vi "GA_FitnessFunction.vi"(1 "Init? (F)":bool, 2 "ClassifierClass.lvclass":refnum<class "ClassifierClass.lvclass">, 3 "Phenotype":i8[](array[numeric])) -> (0 "Fitness":dbl)   [LabVIEW 2016, in "GA.lvlib"]
uses:
  GA.lvlib
  4. Accuracy Assessment for EEG Classification/_vlib/ClassifierClass.lvclass
  4. Accuracy Assessment for EEG Classification/_vlib/CU_DataTypes.ctl
  4. Accuracy Assessment for EEG Classification/Classifier.lvlib
panel:
  # "This VI is a part of BCI Design library, http://www.ru-bci.org \nCopyright © 2020, Sotnikov Peter, All rights reserved. License: GNU GPLv3"
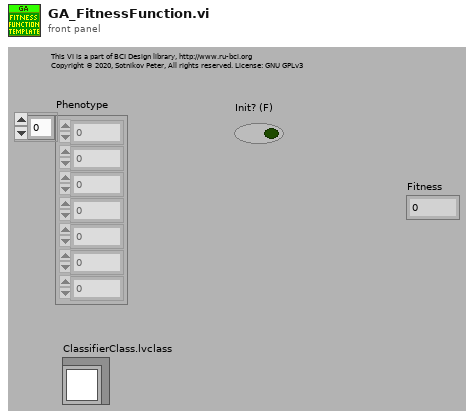
[diagram p1: front panel]
types:
  T1 = typedef "Classifier.lvlib/CU_DataTypes.ctl" = enum16{"Training Data", "Test Data", "Training Data (cross-check)", "Test Data (cross-check)"}
  T2 = typedef "Classifier.lvlib/CU_ClassifierTypes.ctl" = enum16{"Multilayer perceptron", "k NN Classifier", "SVM Committee", "Mahalanobis distance", "SVM Classifier"}
  T3 = typedef "IMAQ Classifier Session.ctl" = refnum<k1>
  T4 = typedef "NILabs_MLT.lvlib/ml_BP_Project.ctl" = cluster{"Training Data":T5, "Normalize Info":T6, "3-layer NN":T7, "Ternimal Condition":T8}
  T5 = typedef "NILabs_MLT.lvlib/ml_BP_Data.ctl" = cluster{"dim in":i32, "dim out":i32, "# samples":i32, "Input":dbl[][], "Output":dbl[][]}
  T6 = typedef "NILabs_MLT.lvlib/ml_BP_Normalize Data.ctl" = cluster{"input min":dbl[], "input max":dbl[], "output min":dbl[], "output max":dbl[]}
  T7 = typedef "NILabs_MLT.lvlib/ml_BP_3layer Feedforward.ctl" = cluster{"# input neuron ":i32, "# hidden neuron":i32, "# output neuron":i32, "Weight (I->H)":dbl[][], "Weight (H->O)":dbl[][], "Output":dbl[][], "Hidden Out":dbl[][], "Derivation Output":dbl[][], "Derivation Hidden":dbl[][], "dw (I->H)":dbl[][], "dw (H->O)":dbl[][]}
  T8 = typedef "NILabs_MLT.lvlib/ml_BP_Terminal Condition.ctl" = cluster{"min MSE":dbl, "min delta MSE":dbl, "min step length":dbl, "max iteration":dbl}
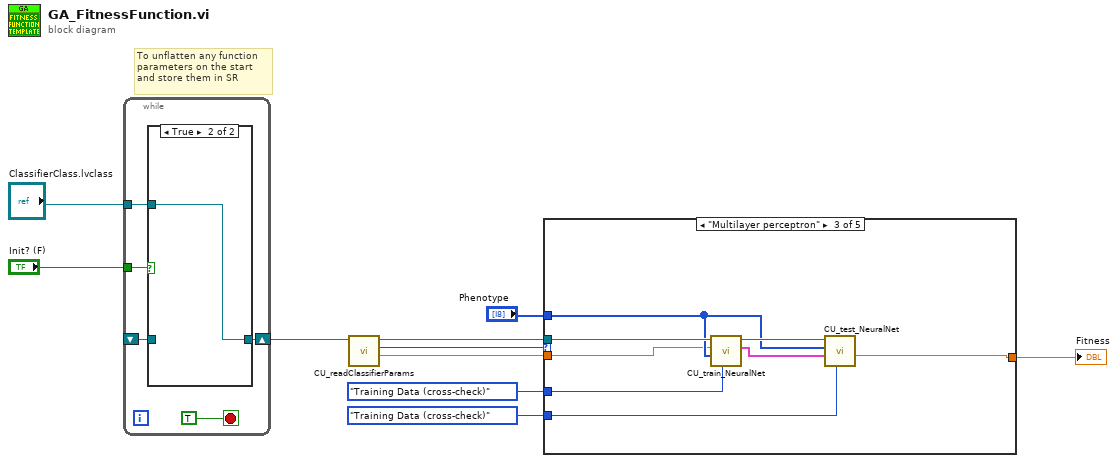
[diagram p0: block diagram]
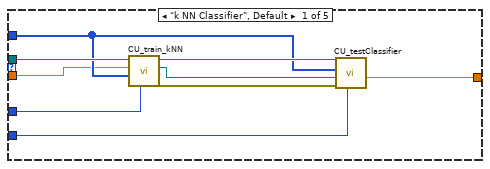
[diagram p2: hidden frame]
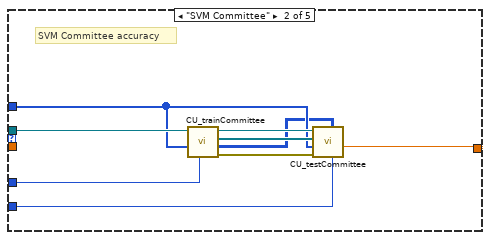
[diagram p3: hidden frame]
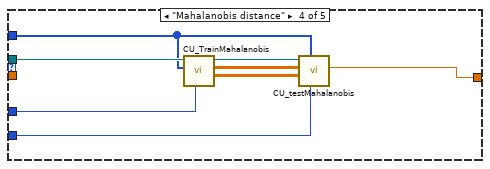
[diagram p4: hidden frame]
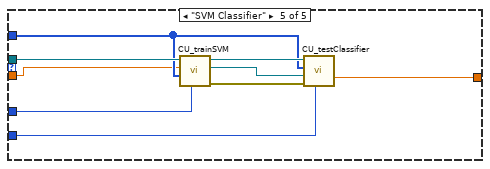
[diagram p5: hidden frame]
diagram:
  # "To unflatten any function\nparameters on the start\nand store them in SR"
  n1 = while {
    tunnel: "ClassifierClass.lvclass" -> [w13]
    tunnel: "Init? (F)" -> [w14]
    shift-right: [w12] -> w7
    shift-left: _ -> [w11]
    stop <- TRUE stop-if-true
    n2 = case shown="True" w14 {
      tunnel: w13 -> [_ w17]
      tunnel: [w16 w17] -> w12
      tunnel: w11 -> [w16 _]
      frame False {
      }
      frame True {
      }
    }
  }
  n3 = call-dynamic "CU_readClassifierParams.vi"("ClassifierClass in"=w7) -> ("Classifier Metaparameter out"=w1:dbl, "ClassifierType out"=w5:T2, "ClassifierClass out"=w6:refnum<class "ClassifierClass.lvclass">)  [unwired: 7 in, 1 out]
  n4 = case shown="\"Multilayer perceptron\"" w5 {
    tunnel: w6 -> [w26 w35 w43 w51 w60]
    tunnel: [w21 w30 w39 w45 w57] -> w2
    tunnel: "Phenotype" -> [w23 w31 w40 w48 w53]
    tunnel: CU_DataTypes."Training Data (cross-check)" ("DataTypes") -> [w20 w28 w38 w50 w59]
    tunnel: CU_DataTypes."Training Data (cross-check)" ("DataTypes") -> [w19 w27 w37 w44 w55]
    tunnel: w1 -> [w18 _ w36 _ w52]
    frame "k NN Classifier", Default {
      n5 = call "CU_train_kNN.vi"("DataTypes"=w20, "Indices"=w23, "k value"=w18, "ClassifierClass in"=w26) -> ("error out"=w22:errorcluster, "Classifier Session out"=w24:T3, "ClassifierClass out"=w25:refnum<class "ClassifierClass.lvclass">)  [unwired: 5 in]
      n6 = call "CU_testClassifier.vi"("DataTypes"=w19, "error in"=w22, "Classifier Session Ref"=w24, "Indices"=w23, "ClassifierClass in"=w25) -> ("Accuracy"=w21:dbl)  [unwired: 3 in, 3 out]
    }
    frame "SVM Committee" {
      # "SVM Committee accuracy"
      n7 = call "CU_trainCommittee.vi"("DataTypes"=w28, "Indices"=w31, "ClassifierClass in"=w35) -> ("error out"=w33:errorcluster, "Classification Distribution"=w29:i32[][][], "Classifier Refs out"=w32:T3[], "ClassifierClass out"=w34:refnum<class "ClassifierClass.lvclass">)  [unwired: 5 in]
      n8 = call "CU_testCommittee.vi"("ClassifierClass in"=w34, "Classifier Refs in"=w32, "Indices"=w31, "error in"=w33, "Classification Distribution"=w29, "DataTypes"=w27) -> ("Accuracy"=w30:dbl)  [unwired: 3 out]
    }
    frame "Multilayer perceptron" {
      n9 = call "CU_train_NeuralNet.vi"("DataTypes"=w38, "Indices"=w40, "# of hidden neuron"=w36, "ClassifierClass in"=w43) -> ("ANN out"=w41:T4, "ClassifierClass out"=w42:refnum<class "ClassifierClass.lvclass">)  [unwired: 4 in, 2 out]
      n10 = call "CU_test_NeuralNet.vi"("DataTypes"=w37, "ANN in"=w41, "Indices"=w40, "ClassifierClass in"=w42) -> ("Accuracy"=w39:dbl)  [unwired: 4 in, 3 out]
    }
    frame "Mahalanobis distance" {
      n11 = call "CU_TrainMahalanobis.vi"("DataTypes"=w50, "Indices"=w48, "ClassifierClass in"=w51) -> ("Mean vectors"=w47:dbl[][], "Covariance matricies"=w46:dbl[][][], "ClassifierClass out"=w49:refnum<class "ClassifierClass.lvclass">)  [unwired: 5 in, 1 out]
      n12 = call "CU_testMahalanobis.vi"("DataTypes"=w44, "Indices"=w48, "Mean vectors"=w47, "Covariance matricies"=w46, "ClassifierClass in"=w49) -> ("Accuracy"=w45:dbl)  [unwired: 3 in, 3 out]
    }
    frame "SVM Classifier" {
      n13 = call "CU_trainSVM.vi"("Train Data"=w59, "Indices"=w53, "Nu Value"=w52, "ClassifierClass in"=w60) -> ("error out"=w56:errorcluster, "Classifier Session out"=w54:T3, "ClassifierClass out"=w58:refnum<class "ClassifierClass.lvclass">)  [unwired: 5 in]
      n14 = call "CU_testClassifier.vi"("DataTypes"=w55, "error in"=w56, "Classifier Session Ref"=w54, "Indices"=w53, "ClassifierClass in"=w58) -> ("Accuracy"=w57:dbl)  [unwired: 3 in, 3 out]
    }
  }
  "Fitness" <- w2
